vi "write_acq_time.vi"(8 "error in (no error)":errorcluster, 10 "acq_time":i32, 11 "picoharp in":refnum<class "picoharp.lvclass">) -> (0 "error out":errorcluster, 3 "picoharp out":refnum<class "picoharp.lvclass">)   [LabVIEW 2015, in "picoharp.lvclass"]
uses:
  picoharp.lvclass
  picoharp.lvclass/picoharp.ctl
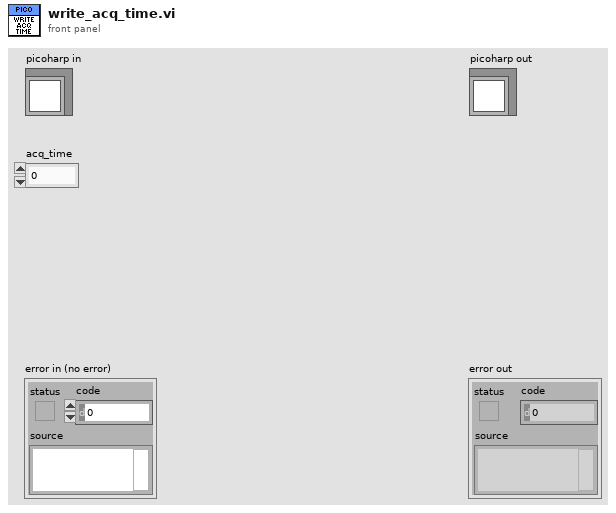
[diagram p1: front panel]
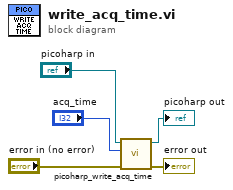
[diagram p0: block diagram]
diagram:
  n1 = call "picoharp_write_acq_time.vi"("error in (no error)"="error in (no error)", "acq_time"="acq_time", "hydraharp in"="picoharp in") -> ("error out"=→"error out":errorcluster, "hydraharp out"=→"picoharp out":refnum<class "picoharp.lvclass">)  [unwired: 7 in]
